vi "Check Chassis Master.vi"(8 "error in (no error)":errorcluster, 11 "Device Item Ref in":T1 format="%.0x") -> (0 "error out":errorcluster, 2 "Master?":bool, 3 "Item Ref out":T1 format="%.0x")   [LabVIEW 2017, in "Chassis TimeSync System Explorer.lvlib"]
uses:
  Chassis TimeSync System Explorer.lvlib
  <vilib>/NI Veristand/Custom Device API/Custom Device Item Ref.ctl
  NationalInstruments.VeriStand.SystemStorage
  Shared/Constants.vi
  <vilib>/NI Veristand/Custom Device API/Custom Device API.lvlib
  Shared/Chassis TimeSync Shared.lvlib
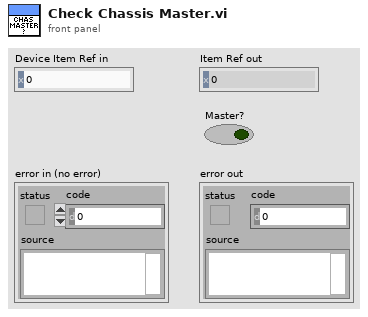
[diagram p1: front panel]
types:
  T1 = typedef "Custom Device API.lvlib/Custom Device Item Ref.ctl" = u64
  T2 = typedef "Custom Device API.lvlib/Custom Device Pointer.ctl" = refnum<k24>
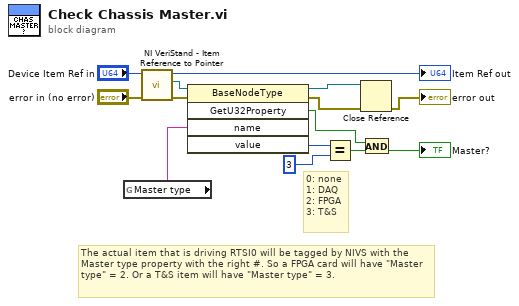
[diagram p0: block diagram]
diagram:
  # "The actual item that is driving RTSI0 will be tagged by NIVS with the Master type property with the right #. So a FPGA card will have \"Master type\" = 2. Or a T&S item will have \"Master type\" = 3."
  # "0: none\n1: DAQ\n2: FPGA\n3: T&S"
  n1 = global read "Constants.vi" "Master type"() -> (w14:string)
  n2 = call <vilib>:"NI VeriStand - Item Reference to Pointer.vi"("error in (no error)"="error in (no error)", "Item Ref in"="Device Item Ref in") -> ("error out"=w6:errorcluster, "Node Pointer"=w5:T2, "Item Ref out"=→"Item Ref out":T1)  [unwired: 6 in, 1 out]
  n3 = invoke class="BaseNodeType" method="GetU32Property"(reference=w5, error in=w6, "name"=w14) -> (reference out=w8:T2, error out=w7:errorcluster, "GetU32Property"=w1:bool, "value"=w11:u32)  [unwired: 2 in, 1 out]
  n4 = Equal?(x=w11, y=u32 3) -> (x = y?=w13:bool)
  n5 = Close Reference(reference=w8, error in (no error)=w7) -> (error out=→"error out":errorcluster)
  n6 = And(x=w1, y=w13) -> (x .and. y?=→"Master?":bool)
